vi "unmake_reg_config_ASIC.vi"(0 "In_reg_value":u32 format="%x") -> (1 "error":bool, 2 "Clip_sel_b":u32, 3 "Ib_clipVb":u32, 4 "Att_en_b":u32, 5 "CompBuf_en_b":bool, 6 "Clip_en_b":bool, 7 "Att_en_b":bool)   [LabVIEW 2009]
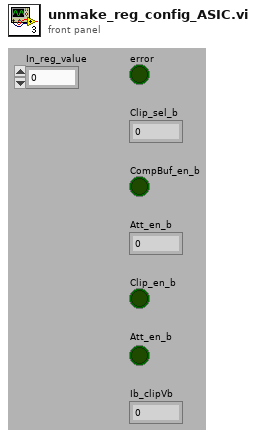
[diagram p1: front panel]
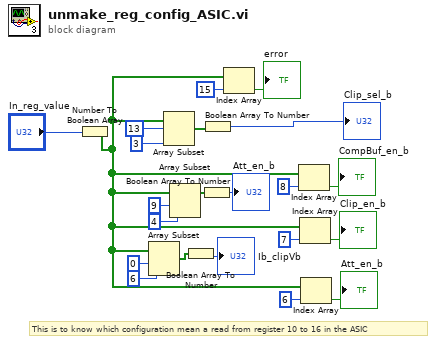
[diagram p0: block diagram]
diagram:
  # "This is to know which configuration mean a read from register 10 to 16 in the ASIC"
  n1 = Number To Boolean Array(number="In_reg_value") -> (Boolean array=w13:bool[])
  n2 = Array Subset(array=w13, index=0, length=6) -> (w18:bool[])
  n3 = Array Subset(array=w13, index=13, length=3) -> (w3:bool[])
  n4 = Array Subset(array=w13, index=9, length=4) -> (w19:bool[])
  n5 = Boolean Array To Number(Boolean array=w18) -> (number=→"Ib_clipVb":u32)
  n6 = Boolean Array To Number(Boolean array=w19) -> (number=→"Att_en_b":u32)
  n7 = Boolean Array To Number(Boolean array=w3) -> (number=→"Clip_sel_b":u32)
  n8 = Index Array(array=w13, index=15) -> (element=→"error":bool)
  n9 = Index Array(array=w13, index=8) -> (element=→"CompBuf_en_b":bool)
  n10 = Index Array(array=w13, index=7) -> (element=→"Clip_en_b":bool)
  n11 = Index Array(array=w13, index=6) -> (element=→"Att_en_b":bool)
